vi "Write I16.vi"(8 "Error In":errorcluster) -> (0 "Error Out":errorcluster)   [LabVIEW 2017, in "Tests.lvlib" / "Writer.lvlib"]
uses:
  Writer.lvlib
  src/LabPack/Public/Writer/Writer.lvclass/Writer.ctl
  src/LabPack/Public/Writer/Private/Handle Error.vi
  src/LabPack/Public/Writer/Public/Status/Read Is Error.vi
  src/LabPack/Public/Writer/Public/Status/Read Status.vi
  src/LabPack/Public/Writer/Public/Status/Read Status Message.vi
  src/LabPack/Public/Utility/Status Code.vi
  <vilib>/Utility/error.llb/Error Cluster From Error Code.vi
  <vilib>/addons/_JKI Toolkits/Caraya/classes/Test/Test.lvclass
  <vilib>/addons/_JKI Toolkits/Caraya/classes/Assert/Assert.lvclass
  src/LabPack/Public/Writer/Writer.lvclass
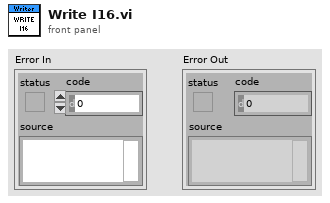
[diagram p1: front panel]
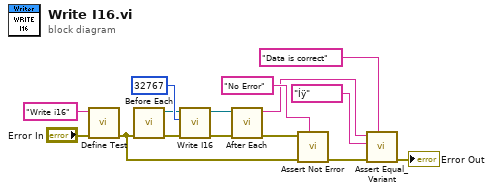
[diagram p0: block diagram]
diagram:
  n1 = call <vilib>:"Define Test.vi"("error in (no error)"="Error In", "Label (VI Title)"="Write i16") -> ("error out"=w3:errorcluster)  [unwired: 9 in]
  n2 = call "Before Each.vi"("Error In"=w3) -> ("Error Out"=w2:errorcluster, "Writer Out"=w1:refnum<class "Writer.lvclass">)  [unwired: 9 in]
  n3 = call "Write I16.vi"("Error In"=w2, "Value"=i16 32767, "Writer In"=w1) -> ("Error Out"=w9:errorcluster, "Writer Out"=w10:refnum<class "Writer.lvclass">)  [unwired: 7 in]
  n4 = call "After Each.vi"("Error In"=w9, "Writer In"=w10) -> ("Error Out"=w11:errorcluster, "Data"=w6:string)  [unwired: 8 in]
  n5 = call <vilib>:"Assert Not Error.vi"("Label"="No Error", "error in (no error)"=w3, "Not Error?"=w11) -> ("error out"=w13:errorcluster)  [unwired: 8 in]
  n6 = call <vilib>:"Assert Equal_Variant.vi"("Label"="Data is correct", "error in (no error)"=w13, "Y"="Íÿ" ("Data"), "X"=w6) -> ("error out"=→"Error Out":errorcluster)  [unwired: 7 in]
